vi "Measure.vi"(6 "PM  results array Refnum":refnum<vi>, 7 "Set Att":bool, 8 "error in (no error)":errorcluster, 9 "Progress Ref":refnum<vi>, 10 "XY Graph Reference":refnum<vi>, 11 "IMD in":refnum<class "IMD.lvclass">) -> (0 "error out":errorcluster, 2 "Results":T1[](array[typedef]), 3 "IMD out":refnum<class "IMD.lvclass">)   [LabVIEW 2020, in "IMD.lvclass"]
uses:
  IMD.lvclass
  C:/Sandbox/RF Bench/Source Code/WiSpry Test Framework/Measurements/Measurement.lvclass
  XML Handler/Controls/Result Cluster.ctl
  Path Control/Paths.ctl
  IMD.lvclass/IMD.ctl
  Instruments/Spectrum Analyzer/Spectrum Analyzer.lvclass/Spectrum Analyzer.ctl
  Measurement.lvclass/Measurement.ctl
  Instruments/Spectrum Analyzer/Controls/Marker Search.ctl
  Instruments/Signal Generator/Signal Generator.lvclass
  Instruments/Spectrum Analyzer/Spectrum Analyzer.lvclass
  Measurement.lvclass
  Path Control/PathControl.lvclass
  XML Handler/XML Handler.lvclass
  Instruments/Power Meter/Power Meter.lvclass
  <vilib>/Analysis/NI_AALPro.lvlib
panel:
  out "Cal values":cluster{"Name":string, "Value":string}[](array[cluster])
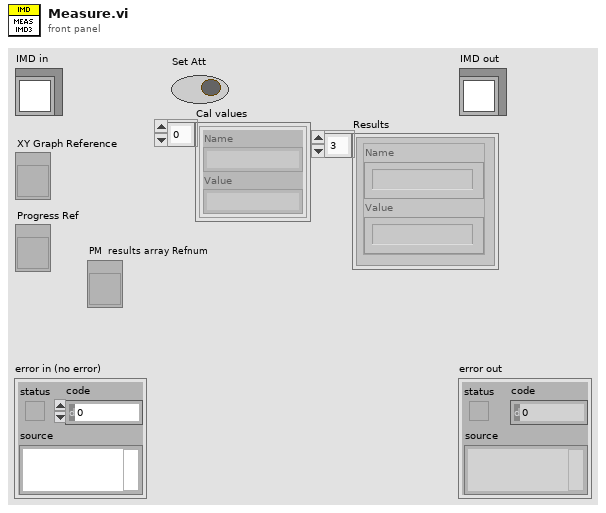
[diagram p1: front panel]
types:
  T1 = typedef "XML Handler.lvclass/Result Cluster.ctl" = cluster{"Name":string, "Value":string}
  T2 = typedef "PathControl.lvclass/Paths.ctl" = enum16{"SigGen 1 -> DUT", "SigGen 2 -> DUT", "SigGen 1 -> PM 1", "SigGen 1 -> PM 2", "DUT -> SA", "DUT -> PM 2", "VSG -> DUT", "SigGen 2 -> PM 1", "SigGen 2 -> PM 2"}
  T3 = typedef "Spectrum Analyzer.lvclass/Marker Search.ctl" = enum16{"Maximum Peak", "Maximum Next", "Maximum Right", "Maximum Left", "Minimum Peak", "Minimum Next", "Minimum Right", "Minimum Left"}
  T4 = typedef "IMD.lvclass/Config info.ctl" = cluster{"RBW":dbl, "VBW ":dbl, "Number of Averages":dbl, "Average On":bool, "Frequency (MHz)":string, "Offset Frequency (MHz)":string, "Power (dBm)":string, "Delta Power (dB)":string, "Uneven IMD":bool, "Loop order":T5, "Stop level":dbl, "IMD2":bool, "IMD3":bool}
  T5 = typedef "IMD.lvclass/Loop order.ctl" = enum16{"Device -> Power -> Frequency -> Offset", "Device -> Frequency -> Power -> Offset"}
  T6 = cluster{"Offset Frequency":dbl, "Mixer Level":dbl}[]
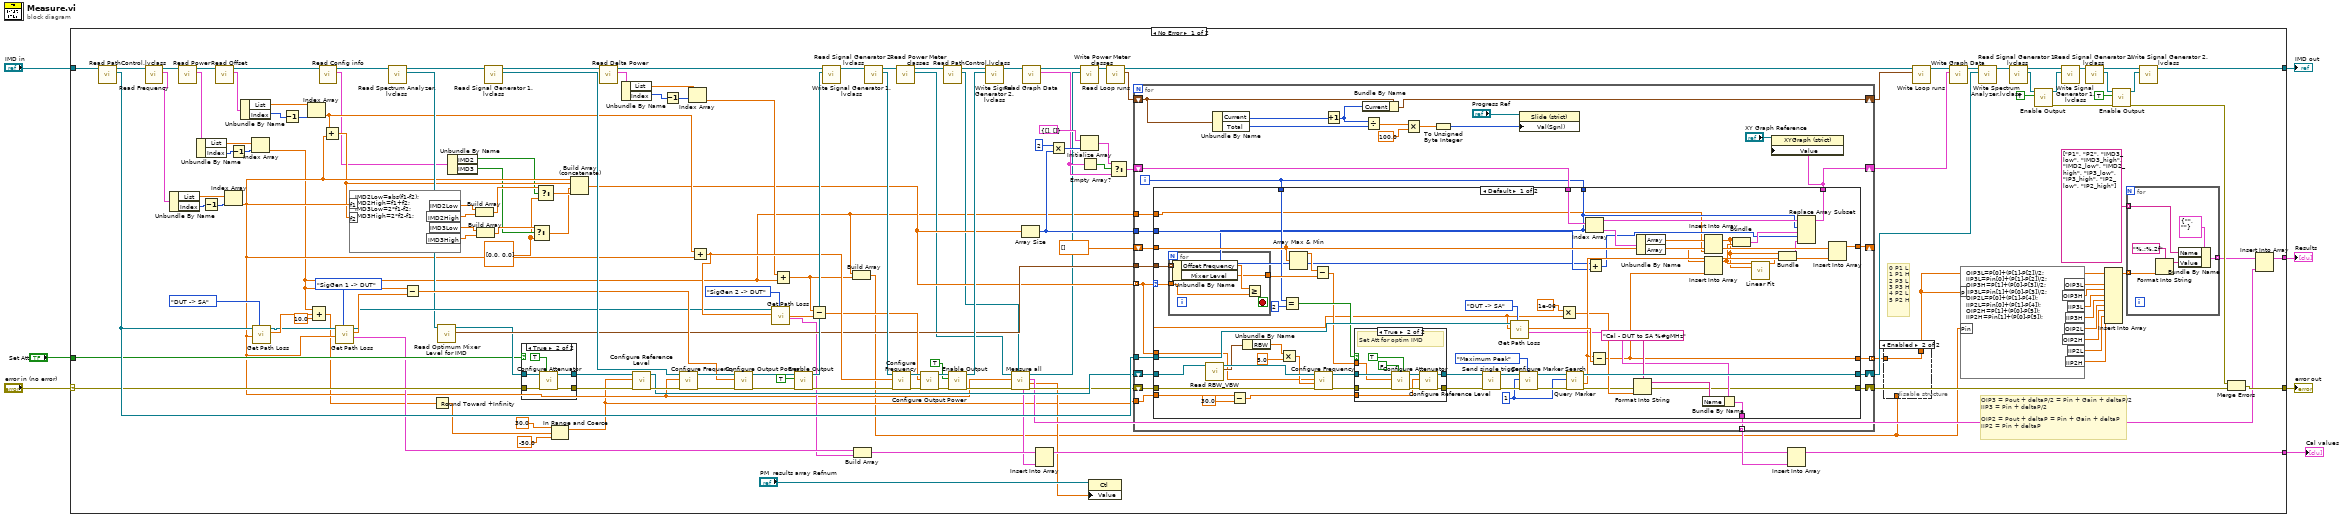
[diagram p0: block diagram]
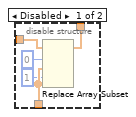
[diagram p2: hidden frame]
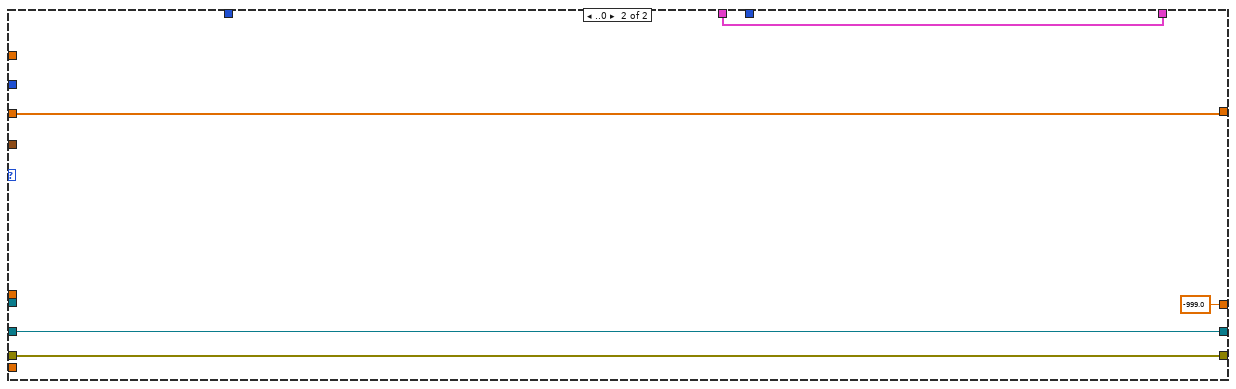
[diagram p5: hidden frame]
diagram:
  n1 = case shown="No Error" "error in (no error)" {
    selector: "error in (no error)" -> [w127 w290]
    tunnel: [w72 w290] -> w6
    tunnel: [w82 w289] -> w4
    tunnel: "IMD in" -> [w160 w289]
    tunnel: [w44 _] -> w3
    tunnel: "Set Att" -> [w91 _]
    tunnel: [w46 _] -> w1
    frame No Error {
      w27 = dbl[] [0.0, 0.0] ("f")
      # "OIP3 = Pout + deltaP/2 = Pin + Gain + deltaP/2\nIIP3 = Pin + deltaP/2\n\nOIP2 = Pout + deltaP = Pin + Gain + deltaP\nIIP2 = Pin + deltaP"
      # "0 P1 L\n1 P1 H\n2 P3 L\n3 P3 H\n4 P2 L\n5 P2 H"
      n2 = call "Read PathControl.lvclass.vi"("Measurements in"=w160) -> ("PathControl.lvclass"=w129:refnum<class "PathControl.lvclass">, "Measurements out"=w159:refnum<class "IMD.lvclass">)  [unwired: 9 in]
      n3 = call "Read Frequency.vi"("IMD in"=w159) -> ("Frequency"=w161:cluster{"List":dbl[], "Index":i32, "Last":bool}, "IMD out"=w136:refnum<class "IMD.lvclass">)  [unwired: 9 in]
      n4 = Unbundle By Name(w161) -> ("List"=w150:dbl[], "Index"=w149:i32)
      n5 = call "Read Power.vi"("IMD in"=w136) -> ("Power"=w131:cluster{"List":dbl[], "Index":i32, "Last":bool}, "IMD out"=w135:refnum<class "IMD.lvclass">)  [unwired: 9 in]
      n6 = Unbundle By Name(w131) -> ("List"=w132:dbl[], "Index"=w133:i32)
      n7 = Decrement(x=w149) -> (x-1=w148:i32)
      n8 = call "Read Offset.vi"("IMD in"=w135) -> ("Offset"=w140:cluster{"List":dbl[], "Index":i32, "Last":bool}, "IMD out"=w32:refnum<class "IMD.lvclass">)  [unwired: 9 in]
      n9 = Index Array(array=w150, index=w148) -> (element=w42:dbl)
      n10 = Decrement(x=w133) -> (x-1=w134:i32)
      n11 = Unbundle By Name(w140) -> ("List"=w141:dbl[], "Index"=w142:i32)
      n12 = Index Array(array=w132, index=w134) -> (element=w16:dbl)
      n13 = call "Get Path Loss.vi"("Path"=Paths."DUT -> SA", "Frequency [Hz]"=w42, "PathControl in"=w129) -> ("Insertion Loss (dB)"=w124:dbl, "PathControl out"=w117:refnum<class "PathControl.lvclass">)  [unwired: 5 in, 2 out]
      n14 = Decrement(x=w142) -> (x-1=w143:i32)
      n15 = Index Array(array=w141, index=w143) -> (element=w90:dbl)
      n16 = Compound Arithmetic op=ADD(w16, w124, 10.0 ("value")) -> (w21:dbl)
      n17 = call "Read Config info.vi"("IMD in"=w32) -> ("Config info"=w30:T4, "IMD out"=w31:refnum<class "IMD.lvclass">)  [unwired: 9 in]
      n18 = Add(x=w90, y=w42) -> (x+y=w41:dbl)
      n19 = call "Get Path Loss.vi"("Path"=Paths."SigGen 1 -> DUT", "Frequency [Hz]"=w42, "PathControl in"=w117) -> ("Parameter"=w51:cluster{"Name":string, "Value":string}, "Insertion Loss (dB)"=w115:dbl, "PathControl out"=w105:refnum<class "PathControl.lvclass">)  [unwired: 5 in, 1 out]
      n20 = formula code="IMD2Low=abs(f1-f2);\nIMD2High=f1+f2;\nIMD3Low=2*f1-f2;\nIMD3High=2*f2-f1;"("f1"=w42, "f2"=w41) -> ("IMD2Low"=w40:dbl, "IMD2High"=w39:dbl, "IMD3Low"=w38:dbl, "IMD3High"=w37:dbl)
      n21 = call "Read Spectrum Analyzer.lvclass.vi"("IMD in"=w31) -> ("Spectrum Analyzer.lvclass"=w94:refnum<class "Spectrum Analyzer.lvclass">, "IMD out"=w130:refnum<class "IMD.lvclass">)  [unwired: 9 in]
      n22 = Subtract(x=w16, y=w115) -> (x-y=w114:dbl)
      n23 = Round Toward +Infinity(x=w21) -> (ceil(x): smallest int >= x=w20:dbl)
      n24 = call "Read Optimum Mixer Level for IMD.vi"("Spectrum Analyzer in"=w94) -> ("Optimum Mixer Level for IMD"=w93:T6, "Spectrum Analyzer out"=w92:refnum<class "Spectrum Analyzer.lvclass">)  [unwired: 9 in]
      n25 = Unbundle By Name(w30) -> ("IMD2"=w29:bool, "IMD3"=w28:bool)
      n26 = Build Array(w40, w39) -> (w35:dbl[])
      n27 = Build Array(w38, w37) -> (w36:dbl[])
      n28 = call "Read Signal Generator 1.lvclass.vi"("IMD in"=w130) -> ("Signal Generator 1.lvclass"=w122:refnum<class "Signal Generator.lvclass">, "IMD out"=w158:refnum<class "IMD.lvclass">)  [unwired: 9 in]
      n29 = case shown="True" w91 {
        tunnel: w127 -> [w168 w174]
        tunnel: [w168 w172] -> w126
        tunnel: [w169 w171] -> w125
        tunnel: w92 -> [w169 w170]
        frame False {
        }
        frame True {
          n30 = call-dynamic "Configure Attenuator.vi"("Auto Attenuator (T)"=TRUE, "error in (no error)"=w174, "Spectrum Analyzer in"=w170) -> ("error out"=w172:errorcluster, "Spectrum Analyzer out"=w171:refnum<class "Spectrum Analyzer.lvclass">)  [unwired: 7 in]
        }
      }
      n31 = Select(t=w36, s=w28, f=w27) -> (s? t:f=w33:dbl[])
      n32 = Select(t=w35, s=w29, f=w27) -> (s? t:f=w34:dbl[])
      n33 = In Range and Coerce(upper limit=30.0, x=w20, lower limit=-50.0 ("Reference Level [dBm]")) -> (coerced(x)=w17:dbl)  [unwired: 1 out]
      n34 = Build Array (concatenate)(w42, w41, w33, w34) -> (w87:dbl[])
      n35 = call "Read Delta Power.vi"("IMD in"=w158) -> ("Delta Power"=w97:cluster{"List":dbl[], "Index":i32, "Last":bool}, "IMD out"=w101:refnum<class "IMD.lvclass">)  [unwired: 9 in]
      n36 = Unbundle By Name(w97) -> ("List"=w100:dbl[], "Index"=w99:i32)
      n37 = call-dynamic "Configure Reference Level.vi"("error in (no error)"=w126, "Reference Level [dBm]"=w17, "Spectrum Analyzer in"=w125) -> ("error out"=w123:errorcluster, "Spectrum Analyzer out"=w95:refnum<class "Spectrum Analyzer.lvclass">)  [unwired: 7 in]
      n38 = Decrement(x=w99) -> (x-1=w98:i32)
      n39 = call-dynamic "Configure Frequency.vi"("error in (no error)"=w123, "Frequency [Hz]"=w42, "Signal Generator in"=w122) -> ("error out"=w121:errorcluster, "Signal Generator out"=w120:refnum<class "Signal Generator.lvclass">)  [unwired: 7 in]
      n40 = Index Array(array=w100, index=w98) -> (element=w96:dbl)
      n41 = Add(x=w90, y=w42) -> (x+y=w106:dbl)
      n42 = call-dynamic "Configure Output Power.vi"("error in (no error)"=w121, "Output Power [dBm]"=w114, "Signal Generator in"=w120) -> ("error out"=w118:errorcluster, "Signal Generator out"=w119:refnum<class "Signal Generator.lvclass">)  [unwired: 7 in]
      n43 = call "Get Path Loss.vi"("Path"=Paths."SigGen 2 -> DUT", "Frequency [Hz]"=w106, "PathControl in"=w105) -> ("Parameter"=w50:cluster{"Name":string, "Value":string}, "Insertion Loss (dB)"=w104:dbl)  [unwired: 5 in, 2 out]
      n44 = Add(x=w96, y=w16) -> (x+y=w15:dbl)
      n45 = call-dynamic "Enable Output.vi"("error in (no error)"=w118, "Output Enable (F)"=TRUE, "Signal Generator in"=w119) -> ("error out"=w108:errorcluster, "Signal Generator out"=w146:refnum<class "Signal Generator.lvclass">)  [unwired: 7 in]
      n46 = Subtract(x=w15, y=w104) -> (x-y=w103:dbl)
      n47 = call "Write Signal Generator 1.lvclass.vi"("Signal Generator 1.lvclass"=w146, "IMD in"=w101) -> ("IMD out"=w147:refnum<class "IMD.lvclass">)  [unwired: 9 in]
      n48 = Build Array(w16, w15) -> (w14:dbl[])
      n49 = Build Array(w51, w50) -> (w49:cluster{"Name":string, "Value":string}[])
      n50 = call "Read Signal Generator 2.lvclass.vi"("IMD in"=w147) -> ("Signal Generator.lvclass"=w109:refnum<class "Signal Generator.lvclass">, "IMD out"=w63:refnum<class "IMD.lvclass">)  [unwired: 9 in]
      n51 = call-dynamic "Configure Frequency.vi"("error in (no error)"=w108, "Frequency [Hz]"=w106, "Signal Generator in"=w109) -> ("error out"=w111:errorcluster, "Signal Generator out"=w110:refnum<class "Signal Generator.lvclass">)  [unwired: 7 in]
      n52 = call-dynamic "Read Power Meter classes.vi"("IMD in"=w63) -> ("Power Meter classes"=w56:refnum<class "Power Meter.lvclass">[], "IMD out"=w54:refnum<class "IMD.lvclass">)  [unwired: 9 in]
      n53 = call-dynamic "Configure Output Power.vi"("error in (no error)"=w111, "Output Power [dBm]"=w103, "Signal Generator in"=w110) -> ("error out"=w113:errorcluster, "Signal Generator out"=w112:refnum<class "Signal Generator.lvclass">)  [unwired: 7 in]
      n54 = call "Read PathControl.lvclass.vi"("Measurements in"=w54) -> ("PathControl.lvclass"=w57:refnum<class "PathControl.lvclass">, "Measurements out"=w53:refnum<class "IMD.lvclass">)  [unwired: 9 in]
      n55 = call-dynamic "Enable Output.vi"("error in (no error)"=w113, "Output Enable (F)"=TRUE, "Signal Generator in"=w112) -> ("error out"=w59:errorcluster, "Signal Generator out"=w144:refnum<class "Signal Generator.lvclass">)  [unwired: 7 in]
      n56 = call "Write Signal Generator 2.lvclass.vi"("Signal Generator.lvclass"=w144, "IMD in"=w53) -> ("IMD out"=w62:refnum<class "IMD.lvclass">)  [unwired: 9 in]
      n57 = call "Measure all.vi"("PathControl in"=w57, "Error In"=w59, "Frequency"=w42, "Power Meter classes"=w56) -> ("Error Out"=w58:errorcluster, "Power readings"=w25:dbl[], "Power results"=w43:T1[], "Power Meter classes"=w55:refnum<class "Power Meter.lvclass">[], "Calibration values"=w48:cluster{"Name":string, "Value":string}[])  [unwired: 3 in]
      n58 = Array Size(array=w87) -> (size(s)=w69:i32)
      n59 = call "Read Graph Data.vi"("IMD in"=w62) -> ("Graph Data"=w64:cluster{"Array":dbl[], "Array":dbl[]}[], "IMD out"=w61:refnum<class "IMD.lvclass">)  [unwired: 9 in]
      n60 = Insert Into Array(array=w49, new element=w48) -> (w47:cluster{"Name":string, "Value":string}[])  [unwired: 1 in]
      n61 = Multiply(x=2, y=w69) -> (x*y=w68:i32)
      n62 = call-dynamic "Write Power Meter classes.vi"("Power Meter classes"=w55, "IMD in"=w61) -> ("IMD out"=w60:refnum<class "IMD.lvclass">)  [unwired: 9 in]
      n63 = Initialize Array(cluster{"Array":dbl[], "Array":dbl[]} {"Array"=[], "Array"=[]} ("element"), w68) -> (w65:cluster{"Array":dbl[], "Array":dbl[]}[])
      n64 = Empty Array?(array=w64) -> (empty?=w67:bool)
      n65 = property class="Ctl"(reference="PM  results array Refnum", "Value"=w25) -> ()  [unwired: 1 in, 2 out]
      n66 = call "Read Loop runs.vi"("Measurements in"=w60) -> ("Loop runs"=w154:cluster{"Current":u32, "Total":u32}, "Measurements out"=w153:refnum<class "IMD.lvclass">)  [unwired: 9 in]
      n67 = Select(t=w65, s=w67, f=w64) -> (s? t:f=w66:cluster{"Array":dbl[], "Array":dbl[]}[])
      n68 = for {
        shift-right: [w205] -> w73
        shift-left: w58 -> [w208]
        tunnel: w129 -> [w206]
        shift-right: [w204] -> w157
        shift-left: w95 -> [w207]
        shift-right: [w184] -> w155
        shift-left: w66 -> [w185]
        shift-right: [w188] -> w151
        shift-left: w154 -> [w187]
        tunnel: w87 -> [w197] mode=indexing
        tunnel: w93 -> [w203]
        shift-right: [w202] -> _
        shift-left: dbl[] [] -> [w201]
        tunnel: w16 -> [w181]
        tunnel: [w200] -> w89 mode=indexing
        tunnel: w17 -> [w199]
        tunnel: w69 -> [w183]
        tunnel: [w198] -> w52 mode=indexing
        i -> [w182]
        n69 = case shown="Default" w197 {
          tunnel: w208 -> [w266 w287]
          tunnel: w207 -> [w265 w286]
          tunnel: w206 -> [w259 _]
          tunnel: [w225 w287] -> w205
          tunnel: [w250 w286] -> w204
          tunnel: w203 -> [w249 _]
          tunnel: [w248 w288] -> w202
          tunnel: w201 -> [w246 w288]
          tunnel: [w210 -999.0] -> w200
          tunnel: w199 -> [w236 _]
          tunnel: w197 -> [w231 _]
          tunnel: [w228 _] -> w198
          tunnel: w182 -> [w227 _]
          tunnel: w185 -> [w224 w284]
          tunnel: [w223 w284] -> w184
          tunnel: w183 -> [w222 _]
          tunnel: w182 -> [w221 _]
          tunnel: w181 -> [w211 _]
          frame Default {
            w252 = u32 1 ("Marker Number (1)")
            n70 = for {
              tunnel: w249 -> [w283] mode=indexing
              tunnel: w231 -> [w281]
              tunnel: [w279] -> w244
              stop <- w280 stop-if-true
              n71 = Unbundle By Name(w283) -> ("Offset Frequency"=w282:dbl, "Mixer Level"=w279:dbl)
              n72 = Greater Or Equal?(x=w282, y=w281) -> (x >= y?=w280:bool)
            }
            n73 = call "Read RBW_VBW.vi"("Spectrum Analyzer in"=w265) -> ("RBW/VBW"=w263:cluster{"RBW":dbl, "VBW":dbl}, "Spectrum Analyzer out"=w264:refnum<class "Spectrum Analyzer.lvclass">)  [unwired: 9 in]
            n74 = Subtract(x=w236, y=30.0) -> (x-y=w209:dbl)
            n75 = Unbundle By Name(w263) -> ("RBW"=w262:dbl)
            n76 = Multiply(x=w262, y=5.0) -> (x*y=w260:dbl)
            n77 = Equal?(x=w227, y=2) -> (x = y?=w242:bool)
            n78 = Array Max & Min(array=w246) -> (max value=w245:dbl)  [unwired: 3 out]
            n79 = Subtract(x=w245, y=w244) -> (x-y=w241:dbl)
            n80 = call-dynamic "Configure Frequency.vi"("error in (no error)"=w266, "Span/Stop Frequency [Hz]"=w260, "Center/Start Frequency [Hz]"=w231, "Spectrum Analyzer in"=w264) -> ("error out"=w240:errorcluster, "Spectrum Analyzer out"=w239:refnum<class "Spectrum Analyzer.lvclass">)  [unwired: 6 in]
            n81 = case shown="True" w242 {
              tunnel: w241 -> [_ w276]
              tunnel: w240 -> [w267 w277]
              tunnel: w239 -> [w268 w278]
              tunnel: [w268 w273] -> w238
              tunnel: [w267 w275] -> w237
              tunnel: w209 -> [_ w271]
              frame False {
              }
              frame True {
                # "Set Att for optim IMD"
                n82 = call-dynamic "Configure Attenuator.vi"("Use Eletronic Attenuator (F)"=TRUE ("Auto Attenuator (T)"), "Auto Attenuator (T)"=FALSE, "error in (no error)"=w277, "Attenuator (dB)"=w276, "Spectrum Analyzer in"=w278) -> ("error out"=w272:errorcluster, "Spectrum Analyzer out"=w274:refnum<class "Spectrum Analyzer.lvclass">)  [unwired: 5 in]
                n83 = call-dynamic "Configure Reference Level.vi"("error in (no error)"=w272, "Reference Level [dBm]"=w271, "Spectrum Analyzer in"=w274) -> ("error out"=w275:errorcluster, "Spectrum Analyzer out"=w273:refnum<class "Spectrum Analyzer.lvclass">)  [unwired: 7 in]
              }
            }
            n84 = call-dynamic "Send single trigger.vi"("error in (no error)"=w237, "Spectrum Analyzer in"=w238) -> ("error out"=w257:errorcluster, "Spectrum Analyzer out"=w256:refnum<class "Spectrum Analyzer.lvclass">)  [unwired: 8 in]
            n85 = call "Get Path Loss.vi"("Path"=Paths."DUT -> SA", "Frequency [Hz]"=w231, "PathControl in"=w259) -> ("Parameter"=w229:cluster{"Name":string, "Value":string}, "Insertion Loss (dB)"=w251:dbl)  [unwired: 5 in, 2 out]
            n86 = call-dynamic "Configure Marker Search.vi"("Marker Search (Max Peak)"=Marker_Search."Maximum Peak", "error in (no error)"=w257, "Marker Number (1)"=w252, "Spectrum Analyzer in"=w256) -> ("error out"=w254:errorcluster, "Spectrum Analyzer out"=w253:refnum<class "Spectrum Analyzer.lvclass">)  [unwired: 6 in]
            n87 = Multiply(x=1e-06, y=w231) -> (x*y=w230:dbl)
            n88 = call-dynamic "Query Marker.vi"("error in (no error)"=w254, "Marker Number (1)"=w252, "Spectrum Analyzer in"=w253) -> ("error out"=w226:errorcluster, "Marker Level"=w247:dbl, "Spectrum Analyzer out"=w250:refnum<class "Spectrum Analyzer.lvclass">)  [unwired: 5 in, 1 out]
            n89 = Index Array(array=w224, index=w221) -> (element=w220:cluster{"Array":dbl[], "Array":dbl[]})
            n90 = Add(x=w221, y=w222) -> (x+y=w212:i32)
            n91 = Subtract(x=w247, y=w251) -> (x-y=w210:dbl)
            n92 = Format Into String(format string="Cal - DUT to SA %#gMHz" ("Name"), error in=w226, w230) -> (resulting string=w234:string, error out=w225:errorcluster)  [unwired: 1 in]
            n93 = Unbundle By Name(w220) -> ("Array"=w219:dbl[], "Array"=w218:dbl[])
            n94 = Bundle By Name(cluster=w229, "Name"=w234) -> (w228:cluster{"Name":string, "Value":string})
            n95 = Insert Into Array(array=w219, new element=w211) -> (w213:dbl[])  [unwired: 1 in]
            n96 = Insert Into Array(array=w218, new element=w210) -> (w214:dbl[])  [unwired: 1 in]
            n97 = Bundle("Array"=w213, "Array"=w214) -> (w217:cluster{"Array":dbl[], "Array":dbl[]})  [unwired: 1 in]
            n98 = call <vilib>:"Linear Fit.vi"("Y"=w214, "X"=w213) -> ("Best Linear Fit"=w216:dbl[])  [unwired: 9 in, 4 out]
            n99 = Bundle("Array"=w213, "Best Linear Fit"=w216) -> (w215:cluster{"Array":dbl[], "Best Linear Fit":dbl[]})  [unwired: 1 in]
            n100 = Replace Array Subset(array=w224, new element #1=w217, index #1=w221, new element #2=w215, index #2=w212) -> (w223:cluster{"Array":dbl[], "Array":dbl[]}[])
            n101 = Insert Into Array(array=w246, new element=w247) -> (w248:dbl[])  [unwired: 1 in]
          }
          frame ..0 {
          }
        }
        n102 = Unbundle By Name(w187) -> ("Current"=w196:u32, "Total"=w194:u32)
        n103 = Increment(x=w196) -> (x+1=w195:u32)
        n104 = Bundle By Name(cluster=w187, "Current"=w195) -> (w188:cluster{"Current":u32, "Total":u32})
        n105 = Divide(x=w195, y=w194) -> (x/y=w193:dbl)
        n106 = Multiply(x=w193, y=100.0) -> (x*y=w192:dbl)
        n107 = To Unsigned Byte Integer(number=w192) -> (unsigned 8bit integer=w190:u8)
        n108 = property class="Slide (strict)"(reference="Progress Ref", "Val(Sgnl)"=w190) -> ()  [unwired: 1 in, 2 out]
        n109 = property class="XYGraph (strict)"(reference="XY Graph Reference", "Value"=w184) -> ()  [unwired: 1 in, 2 out]
      }
      n110 = Insert Into Array(array=w47, new element=w52) -> (w46:cluster{"Name":string, "Value":string}[])  [unwired: 1 in]
      n111 = disable-structure shown="Enabled" {
        disable-tunnel: w89 -> [w166 w167]
        disable-tunnel: [w165 w167] -> w88
        disable-tunnel: w14 -> [w164 _]
        frame Disabled {
          n112 = Replace Array Subset(array=w166, new element #1=w164, index #1=0 ("index"), new element #2=w164, index #2=1 ("index")) -> (w165:dbl[])
        }
        frame Enabled {
        }
      }
      n113 = call "Write Loop runs.vi"("Loop runs"=w151, "Measurements in"=w153) -> ("Measurements out"=w152:refnum<class "IMD.lvclass">)  [unwired: 9 in]
      n114 = call "Write Graph Data.vi"("Graph Data"=w155, "IMD in"=w152) -> ("IMD out"=w156:refnum<class "IMD.lvclass">)  [unwired: 9 in]
      n115 = formula code="OIP3L=P[0]+(P[1]-P[2])/2;\nIIP3L=Pin[0]+(P[1]-P[2])/2;\nOIP3H=P[1]+(P[0]-P[3])/2;\nIIP3L=Pin[1]+(P[0]-P[3])/2;\nOIP2L=P[0]+(P[1]-P[4]);\nIIP2L=Pin[0]+(P[1]-P[4]);\nOIP2H=P[1]+(P[0]-P[5]);\nIIP2H=Pin[1]+(P[0]-P[5]);"("P"=w88, "Pin"=w14) -> ("OIP3L"=w8:dbl, "OIP3H"=w9:dbl, "OIP2L"=w24:dbl, "OIP2H"=w23:dbl, "IIP3L"=w10:dbl, "IIP3H"=w11:dbl, "IIP2L"=w13:dbl, "IIP2H"=w12:dbl)
      n116 = call "Write Spectrum Analyzer.lvclass.vi"("Spectrum Analyzer.lvclass"=w157, "IMD in"=w156) -> ("IMD out"=w83:refnum<class "IMD.lvclass">)  [unwired: 9 in]
      n117 = call "Read Signal Generator 1.lvclass.vi"("IMD in"=w83) -> ("Signal Generator 1.lvclass"=w76:refnum<class "Signal Generator.lvclass">, "IMD out"=w86:refnum<class "IMD.lvclass">)  [unwired: 9 in]
      n118 = call-dynamic "Enable Output.vi"("Output Enable (F)"=TRUE, "Signal Generator in"=w76) -> ("error out"=w75:errorcluster, "Signal Generator out"=w79:refnum<class "Signal Generator.lvclass">)  [unwired: 8 in]
      n119 = call "Write Signal Generator 1.lvclass.vi"("Signal Generator 1.lvclass"=w79, "IMD in"=w86) -> ("IMD out"=w85:refnum<class "IMD.lvclass">)  [unwired: 9 in]
      n120 = call "Read Signal Generator 2.lvclass.vi"("IMD in"=w85) -> ("Signal Generator.lvclass"=w78:refnum<class "Signal Generator.lvclass">, "IMD out"=w84:refnum<class "IMD.lvclass">)  [unwired: 9 in]
      n121 = Insert Into Array(array=w88, new element #1=w8, new element #2=w9, new element #3=w10, new element #4=w11, new element #5=w24, new element #6=w23, new element #7=w13, new element #8=w12) -> (w138:dbl[])  [unwired: 1 in]
      n122 = call-dynamic "Enable Output.vi"("error in (no error)"=w75, "Output Enable (F)"=TRUE, "Signal Generator in"=w78) -> ("error out"=w74:errorcluster, "Signal Generator out"=w77:refnum<class "Signal Generator.lvclass">)  [unwired: 7 in]
      n123 = for {
        tunnel: w138 -> [w177] mode=indexing
        tunnel: string[] ["P1", "P2", "IMD3_low", "IMD3_high", "IMD2_low", "IMD2_high", "IP3_low", "IP3_high", "IP2_low", "IP2_high"] -> [w179] mode=indexing
        tunnel: [w175] -> w45 mode=indexing
        n124 = Format Into String(format string="%.;%.2f", w177) -> (resulting string=w176:string)  [unwired: 2 in, 1 out]
        n125 = Bundle By Name(cluster=T1 {"Name"="", "Value"=""} ("Result Cluster"), "Name"=w179, "Value"=w176) -> (w175:T1)
      }
      n126 = call "Write Signal Generator 2.lvclass.vi"("Signal Generator.lvclass"=w77, "IMD in"=w84) -> ("IMD out"=w82:refnum<class "IMD.lvclass">)  [unwired: 9 in]
      n127 = Merge Errors(w74, w73) -> (w72:errorcluster)
      n128 = Insert Into Array(array=w45, new element=w43) -> (w44:T1[])  [unwired: 1 in]
    }
    frame Error {
    }
  }
  "error out" <- w6
  "IMD out" <- w4
  "Results" <- w3
  "Cal values" <- w1
